vi "Messages.vi"() -> (2 "Messages":string, 3 "Faults Present":bool)   [LabVIEW 2009]
uses:
  Apps/OM State Strings.ctl
panel:
  in  "OM State Strings":T1
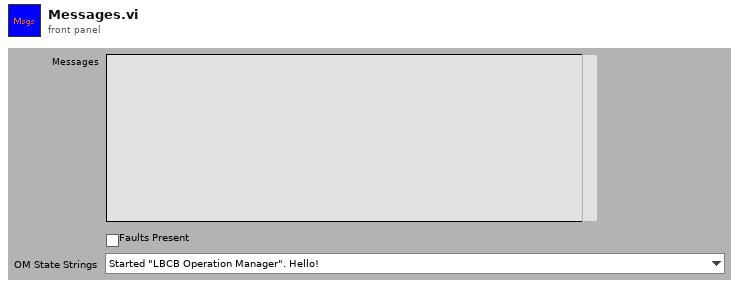
[diagram p1: front panel]
types:
  T1 = typedef "OM State Strings.ctl" = enum16{"Started \"LBCB Operation Manager\". Hello!", "Loading Configuration...", "Setting Up Archiving ...", "Setting Up DAQ Channels...", "Starting Data Acquisition....", "Ready to Auto-Balance Push \"Start Auto-Balance\"...", "Examine Command from last run ...", "Running  Auto-Balance feedback control loop for LBCB 1 ...", "Running  Auto-Balance feedback control loop for LBCB 2 ...", "Ready to start \"Control\" process for LBCB 1. Push \"Control\" button. ", "Ready to start \"Control\" process for LBCB 2. Push \"Control\" button. ", "LBCB 1 under control", "LBCB 2 under control", "Starting control process. Ready to turn on the pump!", "Stopped \"LBCB Operation Manager\". Bye!"}
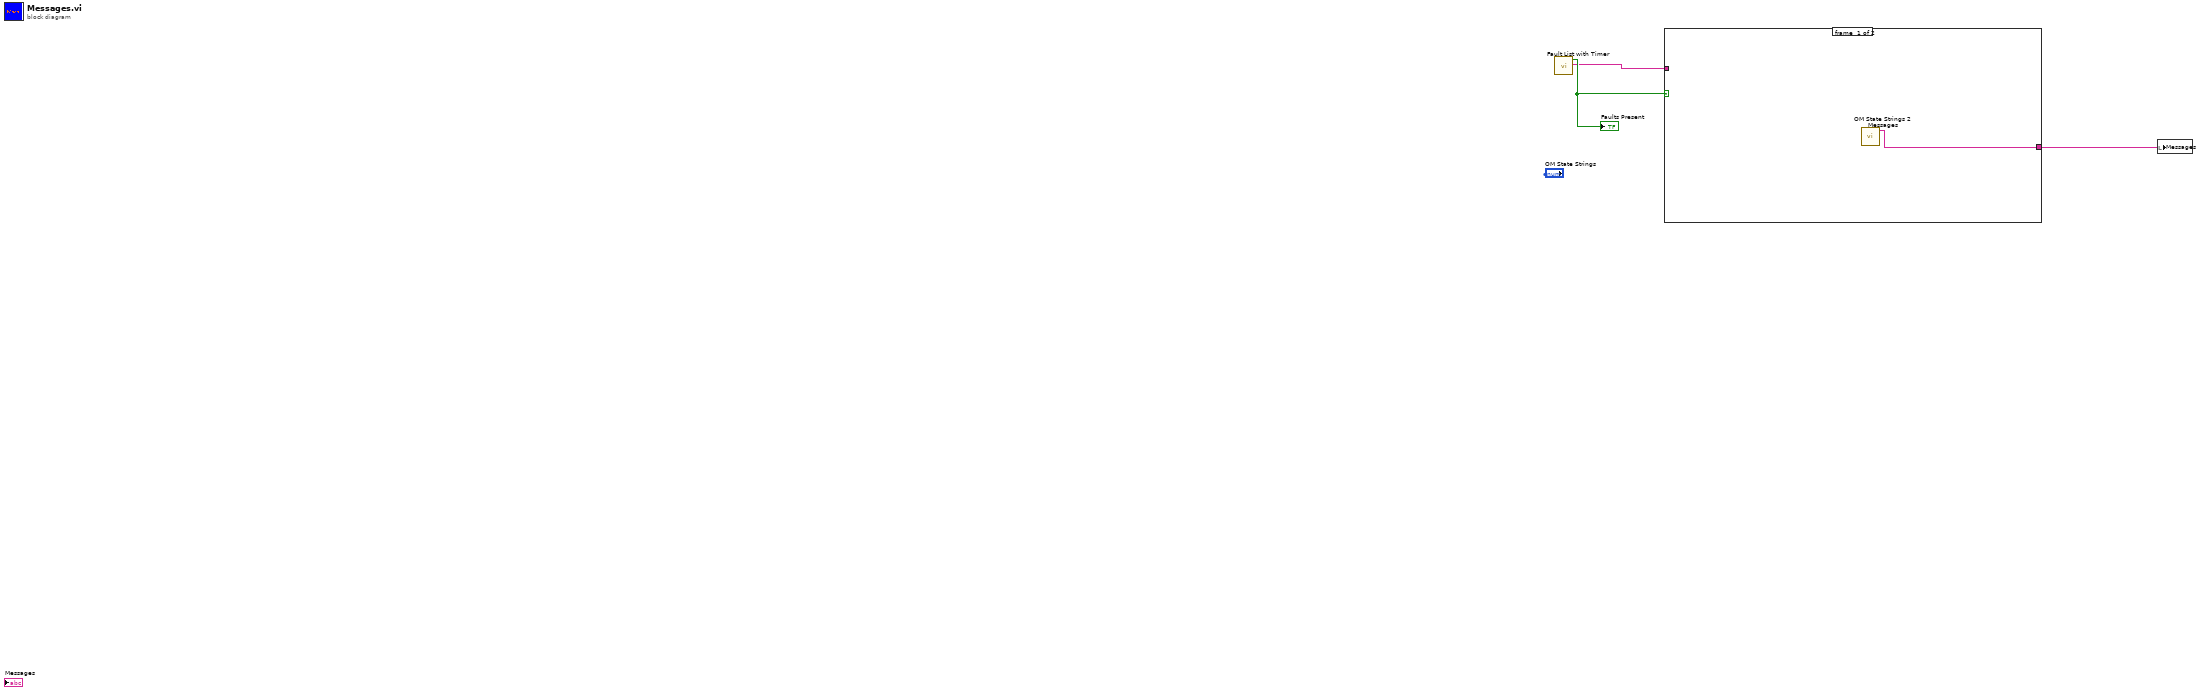
[diagram p0: block diagram]
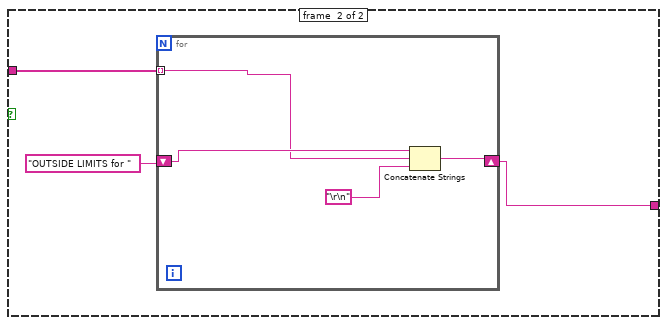
[diagram p2: hidden frame]
diagram:
  n1 = call "Fault List with Timer.vi"() -> ("Fault Strings"=w1:string[], "Faults Present"=w3:bool)  [unwired: 9 in, 1 out]
  "Faults Present" <- w3
  n2 = case shown="True" w3 {
    tunnel: [w4 w6] -> w2
    tunnel: w1 -> [_ w5]
    frame #0 {
      n3 = call "OM State Strings 2 Messages.vi"() -> ("Messages"=w4:string)  [unwired: 11 out]
    }
    frame #1 {
      n4 = for {
        shift-right: [w10] -> w6
        shift-left: "OUTSIDE LIMITS for " -> [w11]
        tunnel: w5 -> [w8] mode=indexing
        n5 = Concatenate Strings(w11, w8, "\r\n" ("string")) -> (w10:string)
      }
    }
  }
  n6 = local write "Messages"(w2) -> ()
